vi "WaveformArrayToVoltageArray.vi"(11 "Waveform Array":waveform(dbl)[](array[waveform])) -> (3 "Average Voltage":dbl[](array[numeric]))   [LabVIEW 2014, in "Analysis.lvlib"]
doc: "Takes a multiple channel waveform array and returns a corresponding array of waveform voltages."
uses:
  Analysis.lvlib
  <vilib>/Analysis/baseanly.llb/Mean (DBL).vi
  <vilib>/Analysis/NI_AALBase.lvlib
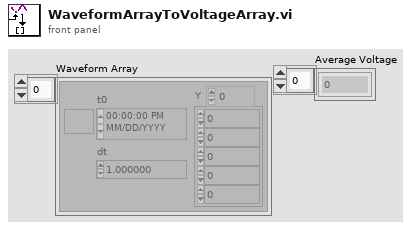
[diagram p1: front panel]
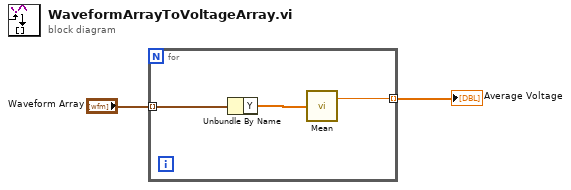
[diagram p0: block diagram]
diagram:
  n1 = for {
    tunnel: "Waveform Array" -> [w5] mode=indexing
    tunnel: [w3] -> w1 mode=indexing
    n2 = Unbundle By Name(w5) -> ("Y"=w4:dbl[])
    n3 = call-poly <vilib>:"Mean.vi"("X"=w4) -> ("mean"=w3:dbl)  [unwired: 1 out]
  }
  "Average Voltage" <- w1
